vi "Main.vi"(8 "error in (no error)":T1) -> ()   [LabVIEW 2019, in "ModuleTemplate.lvlib"]
uses:
  ModuleTemplate.lvlib
  module data.ctl
  Intertarget communication/Status + response + data cluster.ctl
  module state.ctl
  <vilib>/event_ctls.llb/usereventprio.ctl
  5bf6cc24-2521-4779-a80f-885c0f377251.vi
  SubVIs/Shared/Comm GV.vi
  Intertarget communication/CommandResponse communication.lvlib
  SubVIs/Shared/Shared.lvlib
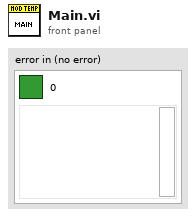
[diagram p1: front panel]
types:
  T1 = cluster{"Boolean Round":bool, "code":i32, "source":string}
  T2 = typedef "CommandResponse communication.lvlib/Status + response + data cluster.ctl" = cluster{"message":string, "response":string, "data":variant}
  T3 = cluster{"message":string, "param":string, "data":variant}
  T4 = typedef "ModuleTemplate.lvlib/module state.ctl" = enum16{"init", "configure", "run", "close"}
  T5 = typedef "ModuleTemplate.lvlib/module data.ctl" = cluster{"dummy":dbl}
  T6 = typedef "usereventprio.ctl" = enum32{"high priority", "normal priority"}
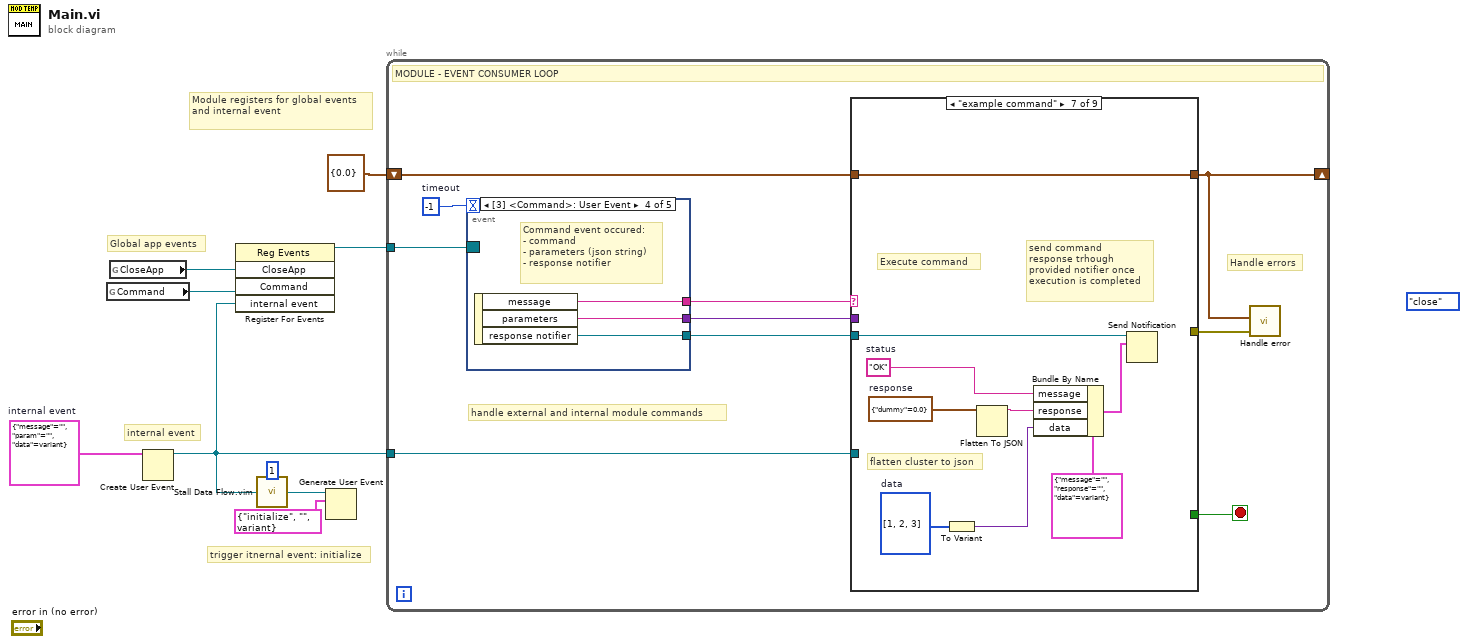
[diagram p0: block diagram]
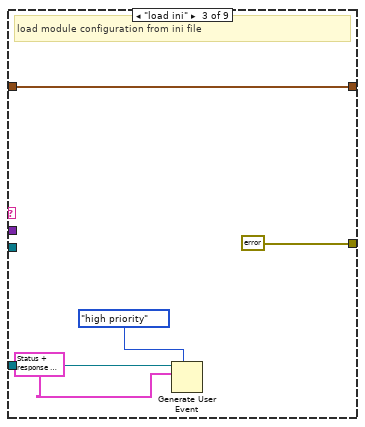
[diagram p4: hidden frame]
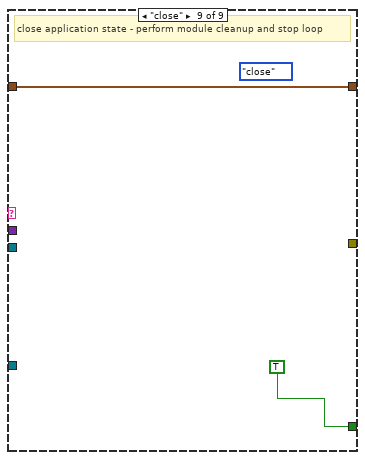
[diagram p9: hidden frame]
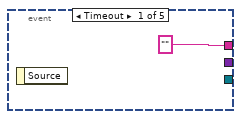
[diagram p10: hidden frame]
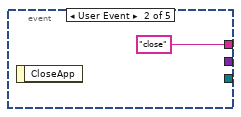
[diagram p11: hidden frame]
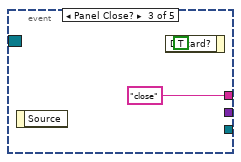
[diagram p12: hidden frame]
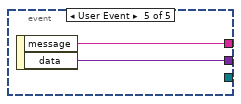
[diagram p13: hidden frame]
diagram:
  w4 = T3 {"message"="", "param"="", "data"=variant}  # internal event
  (unwired) module_state."close" ("module states")
  # "Global app events"
  # "internal event"
  # "trigger itnernal event: initialize"
  # "Module registers for global events\nand internal event"
  n1 = global read "Comm GV.vi" "Command"() -> (w1:refnum<user-event>)
  n2 = global read "Comm GV.vi" "CloseApp"() -> (w2:refnum<user-event>)
  n3 = Create User Event(user event datatype=w4) -> (user event=w7:refnum<user-event>)  [unwired: 1 in, 1 out]
  n4 = register-events(w2, w1, w7) -> (reference out=w9:refnum<event-registration>)  [unwired: 2 in, 1 out]
  n5 = call "Stall Data Flow.vim"("value in"=w7, "milliseconds to wait"=u32 1) -> ("value out"=w6:refnum<user-event>)  [unwired: 1 out]
  n6 = Generate User Event(user event=w6, event data cluster=T2 {"message"="initialize", "response"="", "data"=variant} ("internal command")) -> ()  [unwired: 2 in, 2 out]
  n7 = while {
    tunnel: w9 -> [w19]
    tunnel: w7 -> [w17]
    shift-right: [w11] -> _
    shift-left: T5 {"dummy"=0.0} ("module loopdata") -> [w16]
    stop <- w18 stop-if-true
    w12 = -1  # timeout
    # "Handle errors"
    # "handle external and internal module commands"
    # "MODULE - EVENT CONSUMER LOOP"
    n8 = event shown="[3] <Command>: User Event" {
      selector: w19 -> [_ _ _ _ _]
      dyn-events: _ -> [_ _ _ _ _]
      timeout: w12 -> [_ _ _ _ _]
      tunnel: ["" ("message") "close" "close" w46 w50] -> w15
      tunnel: [_ _ _ w48 w49] -> w14
      tunnel: [_ _ _ w47 _] -> w13
      event Timeout {
        n9 = event-data() -> ()  [unwired: 1 in, 1 out]
      }
      event User Event {
        n10 = event-data() -> ()  [unwired: 1 in, 1 out]
      }
      event Panel Close? {
        n11 = event-data() -> ()  [unwired: 1 in, 1 out]
        n12 = event-data("Discard?"=TRUE) -> ()  [unwired: 1 in, 1 out]
      }
      event User Event {
        # "Command event occured:\n- command\n- parameters (json string)\n- response notifier"
        n13 = event-data() -> ("message"=w46:string, "parameters"=w48:string, "response notifier"=w47:refnum<notifier>)  [unwired: 1 in]
      }
      event User Event {
        n14 = event-data() -> ("message"=w50:string, "data"=w49:variant)  [unwired: 1 in]
      }
    }
    n15 = case shown="\"example command\"" w15 {
      tunnel: [_ _ _ _ _ _ _ _ TRUE] -> w18
      tunnel: w17 -> [_ _ w26 _ _ _ _ _ _]
      tunnel: w16 -> [w20 w21 w25 w27 w28 w29 w38 w39 w40]
      tunnel: [w20 w21 w25 w27 w28 w29 w38 w39 w40] -> w11
      tunnel: w14 -> [_ _ _ _ _ _ _ _ _]
      tunnel: w13 -> [_ _ _ _ _ _ w37 _ _]
      tunnel: [_ _ errorcluster {"status"=FALSE, "code"=0, "source"=""} ("error constant") _ _ _ _ _ _] -> w10
      frame Default {
      }
      frame "----INITIALIZE----" {
      }
      frame "load ini" {
        # "load module configuration from ini file"
        n16 = Generate User Event(priority (normal)=usereventprio."high priority", user event=w26, event data cluster=T2 {"message"="initialize module", "response"="", "data"=variant} ("internal command")) -> ()  [unwired: 1 in, 2 out]
      }
      frame "initialize module" {
        # "initializes module"
      }
      frame "----CONFIGURE----" {
      }
      frame "----RUN----" {
      }
      frame "example command" {
        w31 = i16[] [1, 2, 3]  # data
        w32 = cluster{"dummy":dbl} {"dummy"=0.0}  # response
        w34 = "OK"  # status
        # "Execute command"
        # "send command\nresponse trhough\nprovided notifier once\nexecution is completed"
        # "flatten cluster to json"
        n17 = To Variant(anything=w31) -> (Variant=w30:variant)
        n18 = Flatten To JSON(anything=w32) -> (JSON string=w33:string)  [unwired: 2 in, 1 out]
        n19 = Bundle By Name(cluster=T2 {"message"="", "response"="", "data"=variant} ("notification"), "message"=w34, "response"=w33, "data"=w30) -> (w35:T2)
        n20 = Send Notification(notification=w35, notifier=w37) -> ()  [unwired: 1 in, 2 out]
      }
      frame "----CLEANUP----" {
      }
      frame "close" {
        (unwired) module_state."close" ("module states")
        # "close application state - perform module cleanup and stop loop"
      }
    }
    n21 = call "Handle error.vi"("error in (no error)"=w10, "module loopdata"=w11) -> ()  [unwired: 10 in]
  }
